vi "Insert_Alarm.vi"(1 "备注":string, 2 "连接模式":enum16{"单机", "联网"}(ring), 3 "报警时间":string, 4 "报警类型":string, 5 "报警代码":i32, 6 "报警名称":string) -> (0 "recordset reference":T1)   [LabVIEW 2019]
uses:
  <vilib>/addons/database/Recordset.llb/Rec ObjectReference.ctl
  <vilib>/addons/database/Connection.llb/DB Tools Open Connec (String).vi
  <vilib>/addons/database/Connection.llb/Conn Execute.vi
  <vilib>/addons/database/NI_Database_API.lvlib
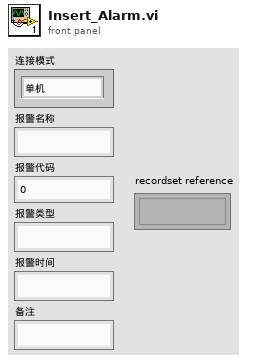
[diagram p1: front panel]
types:
  T1 = typedef "NI_Database_API.lvlib/Rec ObjectReference.ctl" = refnum<k1>
  T2 = typedef "NI_Database_API.lvlib/Conn ObjectReference.ctl" = refnum<k1>
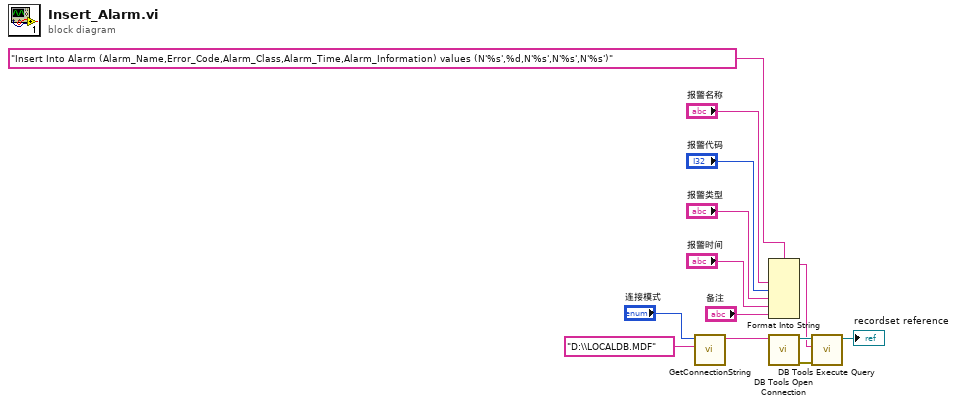
[diagram p0: block diagram]
diagram:
  n1 = call "GetConnectionString.vi"("Database Name"="D:\\LOCALDB.MDF", "连接模式"="连接模式") -> ("连接字符串"=w11:string)  [unwired: 4 in, 1 out]
  n2 = Format Into String(format string="Insert Into Alarm (Alarm_Name,Error_Code,Alarm_Class,Alarm_Time,Alarm_Information) values (N'%s',%d,N'%s',N'%s',N'%s')", "报警名称", "报警代码", "报警类型", "报警时间", "备注") -> (resulting string=w8:string)  [unwired: 2 in, 1 out]
  n3 = call-poly <vilib>:"DB Tools Open Connection.vi"("connection information"=w11) -> ("error out"=w10:errorcluster, "connection reference"=w9:T2)  [unwired: 7 in]
  n4 = call-poly <vilib>:"DB Tools Execute Query.vi"("error in (no error)"=w10, "SQL query"=w8, "connection reference"=w9) -> ("recordset reference"=→"recordset reference":T1)  [unwired: 5 in, 1 out]
